vi "Compare File Binary__ogtk.vi"(4 "error in (no error)":errorcluster, 5 "block size (100000)":i32=100000, 6 "copy file":path, 7 "original file":path) -> (0 "error out":errorcluster, 3 "not equal":bool)   [LabVIEW 2014]
doc: "Compare File Binary.vi - Compares two files to be of the same size and containing the same binary data."
panel:
  # "Compare File Binary.vi\n\nCompares two files to be of the same size and containing the same binary data.\n\nPlease visit http://www.OpenG.org to learn about the\nOpen Source LabVIEW software movement.\n\nNOTICE -- YOU MUST LEAVE THIS NOTICE IN PLACE.  PER THE TERMS OF THE LICENSE BELOW, YOU MAY SUBLICENSE THIS SOFTWARE \nIN ANY WAY THAT DOES NOT CONFLICT WITH THIS LICENSE.\n\n### BSD License (http://www.opensource.org/licenses/bsd-license.php) Begin ###\n\nCopyright (c) 2002, Rolf Kalbermatter <rolf.kalbermatter@citeng.com> \nCopyright (c) 2002-2006, Jim Kring <jim@jimkring.com>\n\nAll rights reserved.\n\nRedistribution and use in source and binary forms, with or without modification, are permitted provided that the following conditions are met:\n\n    * Redistributions of source code must retain the above copyright notice, this list of conditions and the following disclaimer.\n    * Redistributions in binary form must reproduce the above copyright notice, this list of conditions and the following disclaimer in the \n       documentation and/or other materials provided with the distribution.\n    * Neither the name of SciWare, James Kring, Inc., nor the names of its contributors may be used to endorse or promote products derived \n       from this software without specific prior written permission.\n\nTHIS SOFTWARE IS PROVIDED BY THE COPYRIGHT HOLDERS AND CONTRIBUTORS \"AS IS\" AND ANY EXPRESS OR IMPLIED WARRANTIES, \nINCLUDING, BUT NOT LIMITED TO, THE IMPLIED WARRANTIES OF MERCHANTABILITY AND FITNESS FOR A PARTICULAR PURPOSE ARE \nDISCLAIMED. IN NO EVENT SHALL THE COPYRIGHT OWNER OR CONTRIBUTORS BE LIABLE FOR ANY DIRECT, INDIRECT, INCIDENTAL,\n SPECIAL, EXEMPLARY, OR CONSEQUENTIAL DAMAGES (INCLUDING, BUT NOT LIMITED TO, PROCUREMENT OF SUBSTITUTE GOODS OR \nSERVICES; LOSS OF USE, DATA, OR PROFITS; OR BUSINESS INTERRUPTION) HOWEVER CAUSED AND ON ANY THEORY OF LIABILITY, \nWHETHER IN CONTRACT, STRICT LIABILITY, OR TORT (INCLUDING NEGLIGENCE OR OTHERWISE) ARISING IN ANY WAY OUT OF THE USE \nOF THIS SOFTWARE, EVEN IF ADVISED OF THE POSSIBILITY OF SUCH DAMAGE.\n\n### BSD License End ###"
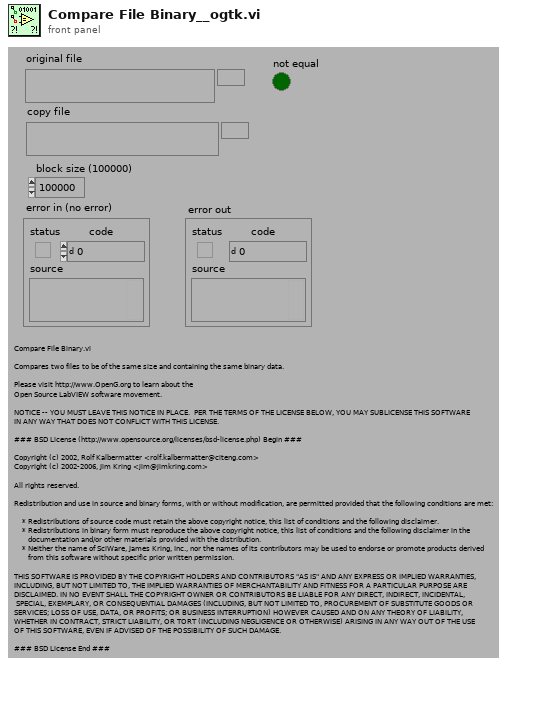
[diagram p1: front panel]
types:
  T1 = enum16{"read/write", "read-only", "write-only", "write-only (truncate)"}
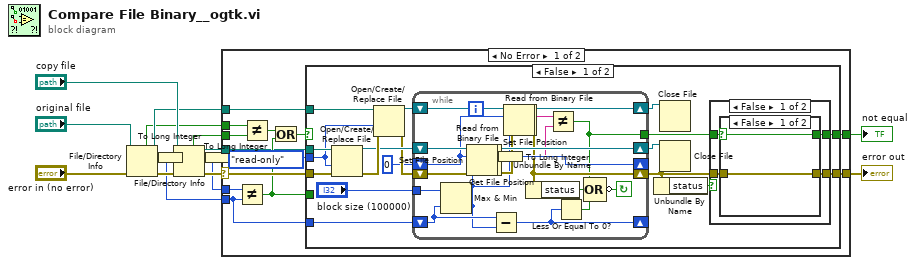
[diagram p0: block diagram]
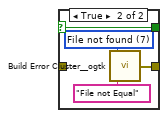
[diagram p2: hidden frame]
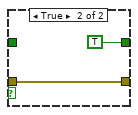
[diagram p3: hidden frame]
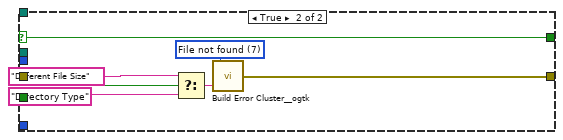
[diagram p4: hidden frame]
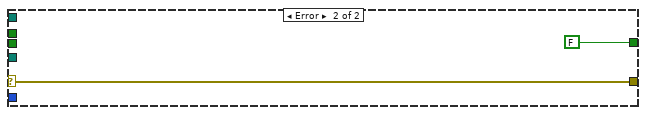
[diagram p5: hidden frame]
diagram:
  n1 = File/Directory Info(path="original file", error in="error in (no error)") -> (path out=w9:path, directory=w4:bool, size=w2:i64, error out=w12:errorcluster)  [unwired: 3 out]
  n2 = To Long Integer(number=w2) -> (32bit integer=w5:i32)
  n3 = File/Directory Info(path="copy file", error in=w12) -> (path out=w10:path, directory=w7:bool, size=w1:i64, error out=w11:errorcluster)  [unwired: 3 out]
  n4 = To Long Integer(number=w1) -> (32bit integer=w6:i32)
  n5 = case shown="No Error" w11 {
    selector: w11 -> [w23 w93]
    tunnel: w6 -> [w28 _]
    tunnel: w5 -> [w18 _]
    tunnel: w7 -> [w27 _]
    tunnel: w4 -> [w26 _]
    tunnel: w10 -> [w21 _]
    tunnel: w9 -> [w20 _]
    tunnel: [w17 w93] -> w8
    tunnel: [w16 FALSE] -> w3
    frame No Error {
      n6 = Not Equal?(x=w28, y=w18) -> (x != y?=w22:bool)
      n7 = Not Equal?(x=w26, y=w27) -> (x != y?=w25:bool)
      n8 = Or(x=w25, y=w22) -> (x .or. y?=w24:bool)
      n9 = case shown="False" w24 {
        selector: w24 -> [_ w85]
        tunnel: w23 -> [w45 _]
        tunnel: w22 -> [_ w88]
        tunnel: w21 -> [w46 _]
        tunnel: w20 -> [w44 _]
        tunnel: T1."read-only" ("open mode (0)") -> [w42 _]
        tunnel: w18 -> [w30 _]
        tunnel: [w34 w91] -> w17
        tunnel: [w32 w85] -> w16
        frame False {
          n10 = Open/Create/Replace File(file path (use dialog)=w46, error in=w45, access (0:read/write)=w42) -> (refnum out=w40:refnum<file>, error out=w43:errorcluster)  [unwired: 3 in, 1 out]
          n11 = Open/Create/Replace File(file path (use dialog)=w44, error in=w43, access (0:read/write)=w42) -> (refnum out=w41:refnum<file>, error out=w39:errorcluster)  [unwired: 3 in, 1 out]
          n12 = while {
            shift-right: [w65] -> w38
            shift-left: w41 -> [w72]
            shift-right: [w69] -> w37
            shift-left: w40 -> [w71]
            shift-right: [w64] -> w35
            shift-left: w39 -> [w70]
            shift-right: [w55] -> _
            shift-left: w30 -> [w57]
            shift-right: [w66] -> _
            shift-left: 0 ("offset") -> [w67]
            tunnel: [w58] -> w33
            tunnel: "block size (100000)" -> [w56]
            stop <- w59 continue-if-true
            n13 = Max & Min(x=w56, y=w57) -> (min(x,y)=w54:i32)  [unwired: 1 out]
            n14 = Set File Position(offset (in bytes) (0)=w67, refnum=w71, error in=w70) -> (refnum out=w53:refnum<file>, error out=w52:errorcluster)  [unwired: 1 in]
            n15 = Read from Binary File(8:w52, 10:w54, 11:w53) -> (0:w50:errorcluster, 2:w63:string, 3:w51:refnum<file>)  [unwired: 3 in, 1 out]
            n16 = Get File Position(4:w50, 7:w51) -> (0:w68:errorcluster, 2:w49:i64, 3:w69:refnum<file>)
            n17 = Subtract(x=w57, y=w54) -> (x-y=w55:i32)
            n18 = To Long Integer(number=w49) -> (32bit integer=w66:i32)
            n19 = Set File Position(offset (in bytes) (0)=w67, refnum=w72, error in=w68) -> (refnum out=w48:refnum<file>, error out=w47:errorcluster)  [unwired: 1 in]
            n20 = Read from Binary File(8:w47, 10:w54, 11:w48) -> (0:w64:errorcluster, 2:w62:string, 3:w65:refnum<file>)  [unwired: 3 in, 1 out]
            n21 = Unbundle By Name(w64) -> ("status"=w61:bool)
            n22 = Not Equal?(x=w62, y=w63) -> (x != y?=w58:bool)
            n23 = Less Or Equal To 0?(x=w55) -> (x <= 0?=w60:bool)
            n24 = Compound Arithmetic op=OR(w58, w61, w60) -> (invert w59:bool)
          }
          n25 = Unbundle By Name(w35) -> ("status"=w36:bool)
          n26 = Close File(refnum=w38) -> ()  [unwired: 1 in, 2 out]
          n27 = Close File(refnum=w37) -> ()  [unwired: 1 in, 2 out]
          n28 = case shown="False" w36 {
            tunnel: w35 -> [w75 w84]
            tunnel: [w74 w84] -> w34
            tunnel: w33 -> [w76 _]
            tunnel: [w73 TRUE] -> w32
            frame False {
              n29 = case shown="False" w76 {
                selector: w76 -> [w77 w79]
                tunnel: w75 -> [w78 _]
                tunnel: [w78 w81] -> w74
                tunnel: [w77 w79] -> w73
                frame False {
                }
                frame True {
                  w82 = 7 items=["No error", "Argument error", "Memory is full", "Out of zone", "End of file", "File already open", "Generic file I/O error", "File not found", "File permission error", "Disk is full", "Duplicate path", "Too many files open", "System feature not enabled", "Resource file not found", "Cannot add resource", "Resource not found", "Image not found", "Image memory error", "Pen does not exist", "Config type invalid", "Config token not found", "Config parse error", "Config memory error", "Bad external code format", "Bad external code offset", "External code not present", "Null window", "Destroy window error", "Null menu", "Print aborted", "Bad print record", "Print driver error", "Windows error during printing", "Memory error during printing", "Print dialog error", "Generic print error", "Invalid device refnum", "Device not found", "Device parameter error", "Device unit error", "Cannot open device", "Device call aborted", "Generic error", "Cancelled by user", "Object ID too low", "Object ID too high", "Object not in heap", "Unknown heap", "Unknown object (invalid DefProc)", "Unknown object (DefProc not in table)", "Message out of range", "Invalid (null) method", "Unknown message", "Manager call not supported", "Bad address", "Network operation in progress", "Network operation timed out", "Connection is busy", "Network attribute not supported", "Network error", "Address in use", "System out of memory", "Connection aborted", "Connection refused", "Not connected", "Already connected", "Connection closed", "Initialization error (interapplication manager)", "Bad occurrence", "Wait on unbound occurrence handler", "Occurrence queue overflow", "Datalog type conflict", "Unused", "Unrecognized type (interapplication manager)", "Memory corrupt", "Failed to make temporary DLL", "Old CIN version", "Drag socket not found", "Failed to load drop-object", "Failed to register OLE object", "Failed to release OLE object", "Format specifier type mismatch", "Unknown format specifier", "Too few format specifiers", "Too many format specifiers", "Scan failed", "Newer CIN version", "Error converting to variant", "Runtime menu error", "Password tampered", "Variant attribute not found", "Incompatible variant data type", "Event data is not available", "Event Store is not present", "Occurrence is not found", "Event Queue is not created", "Event info is not available", "Refnum passed is NULL", "Error retrieving Class GUID", "Error retrieving CoClass GUID", "Error retrieving TypeLib GUID.", "Bad built application magic bytes.", "Specific driver is different from the specific driver associated with the Logical Name.", "There is no session opened to the class driver.", "Max Error", "MAX - Error with config objects", "MAX - Error loading configuration", "MAX - Group not supported"]
                  n30 = call <userlib>:"Build Error Cluster__ogtk.vi"("String to Prepend to source (\"\")"="File not Equal" ("String to Prepend to source (\"\")"), "code"=w82) -> ("error out"=w81:errorcluster)
                }
              }
            }
            frame True {
            }
          }
        }
        frame True {
          w89 = 7 items=["No error", "Argument error", "Memory is full", "Out of zone", "End of file", "File already open", "Generic file I/O error", "File not found", "File permission error", "Disk is full", "Duplicate path", "Too many files open", "System feature not enabled", "Resource file not found", "Cannot add resource", "Resource not found", "Image not found", "Image memory error", "Pen does not exist", "Config type invalid", "Config token not found", "Config parse error", "Config memory error", "Bad external code format", "Bad external code offset", "External code not present", "Null window", "Destroy window error", "Null menu", "Print aborted", "Bad print record", "Print driver error", "Windows error during printing", "Memory error during printing", "Print dialog error", "Generic print error", "Invalid device refnum", "Device not found", "Device parameter error", "Device unit error", "Cannot open device", "Device call aborted", "Generic error", "Cancelled by user", "Object ID too low", "Object ID too high", "Object not in heap", "Unknown heap", "Unknown object (invalid DefProc)", "Unknown object (DefProc not in table)", "Message out of range", "Invalid (null) method", "Unknown message", "Manager call not supported", "Bad address", "Network operation in progress", "Network operation timed out", "Connection is busy", "Network attribute not supported", "Network error", "Address in use", "System out of memory", "Connection aborted", "Connection refused", "Not connected", "Already connected", "Connection closed", "Initialization error (interapplication manager)", "Bad occurrence", "Wait on unbound occurrence handler", "Occurrence queue overflow", "Datalog type conflict", "Unused", "Unrecognized type (interapplication manager)", "Memory corrupt", "Failed to make temporary DLL", "Old CIN version", "Drag socket not found", "Failed to load drop-object", "Failed to register OLE object", "Failed to release OLE object", "Format specifier type mismatch", "Unknown format specifier", "Too few format specifiers", "Too many format specifiers", "Scan failed", "Newer CIN version", "Error converting to variant", "Runtime menu error", "Password tampered", "Variant attribute not found", "Incompatible variant data type", "Event data is not available", "Event Store is not present", "Occurrence is not found", "Event Queue is not created", "Event info is not available", "Refnum passed is NULL", "Error retrieving Class GUID", "Error retrieving CoClass GUID", "Error retrieving TypeLib GUID.", "Bad built application magic bytes.", "Specific driver is different from the specific driver associated with the Logical Name.", "There is no session opened to the class driver.", "Max Error", "MAX - Error with config objects", "MAX - Error loading configuration", "MAX - Group not supported"]
          n31 = Select(t="Different File Size", s=w88, f="Directory Type" ("t")) -> (s? t:f=w90:string)
          n32 = call <userlib>:"Build Error Cluster__ogtk.vi"("String to Prepend to source (\"\")"=w90, "code"=w89) -> ("error out"=w91:errorcluster)
        }
      }
    }
    frame Error {
    }
  }
  "error out" <- w8
  "not equal" <- w3
